vi "setCLMode.vi"(8 "error in":T1, 11 "CL-Mode":i32=-2147483648) -> (0 "error out":T1, 3 "CL-Mode out":i32=-2147483648)   [LabVIEW 2016]
doc: "When \"CL-Mode\" is set to 1, closed loop scanning is active. Note that the CL-Mode can only be changed, when the outputs are deactivated."
uses:
  Controls/Error_Out.ctl
  Files_ASC500/DLL/ASC500_RemoteControlV27.dll
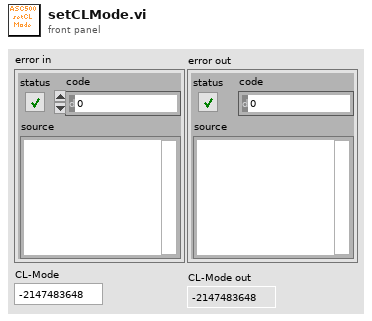
[diagram p1: front panel]
types:
  T1 = typedef "Error_Out.ctl" = errorcluster
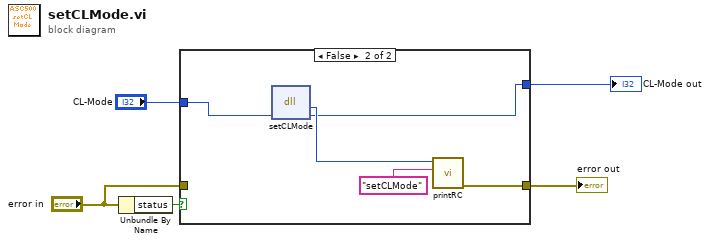
[diagram p0: block diagram]
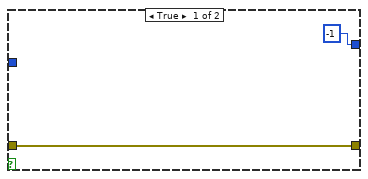
[diagram p2: hidden frame]
diagram:
  n1 = Unbundle By Name("error in") -> ("status"=w3:bool)
  n2 = case shown="False" w3 {
    tunnel: [w7 w11] -> w2
    tunnel: "CL-Mode" -> [_ w12]
    tunnel: "error in" -> [w7 _]
    tunnel: [-1 ("Value") w8] -> w1
    frame True {
    }
    frame False {
      n3 = dll-call lib="G:/SCMOperations/Share/ELE/Produkt Information/ASC500/04 Remote Control/02 development versions/2018Nov06/Files_ASC500/DLL/ASC500_RemoteControlV27.dll" fn="setCLMode"("Value"=w12) -> ("return type"=w10:i32, "Value"=w8:i32)  [unwired: 3 in, 2 out]
      n4 = call "printRC.vi"("additional information"="setCLMode", "RC"=w10) -> ("error out"=w11:T1)  [unwired: 9 in]
    }
  }
  "error out" <- w2
  "CL-Mode out" <- w1
